vi "PhaseCompensation.vi"(1 "error out 2":errorcluster, 2 "Phase  Compensation":dbl) -> (0 "error out":errorcluster)   [LabVIEW 2011]
uses:
  C:/Entwicklungsdaten/Aktuell/Source/LV Source/arcoptix/LCDriver.dll
  Entwicklungsdaten/Aktuell/Source/LV Source/arcoptix/LCDriver.dll
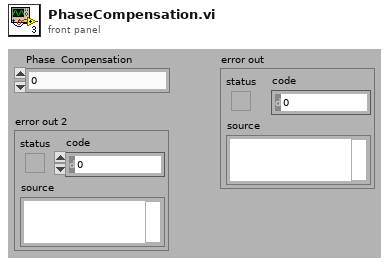
[diagram p1: front panel]
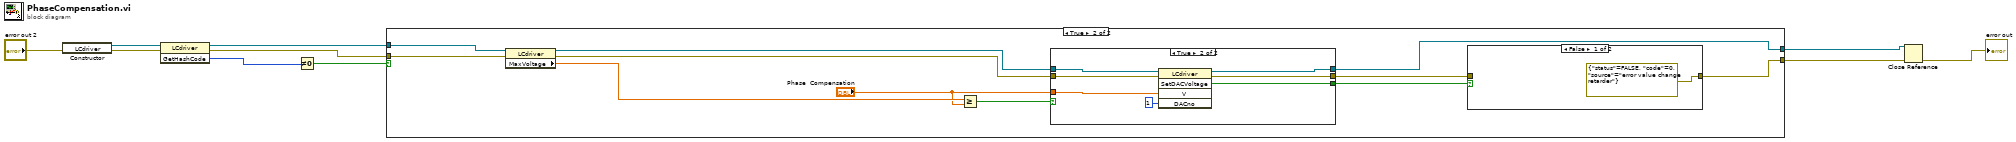
[diagram p0: block diagram]
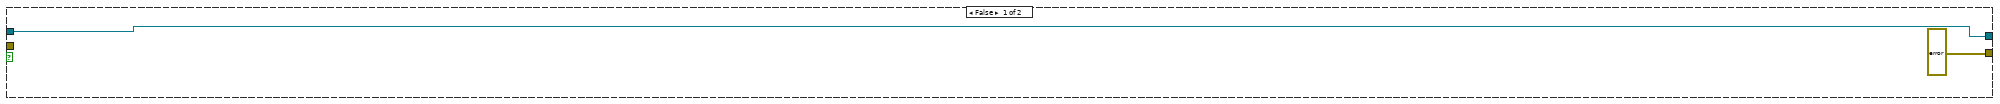
[diagram p2: hidden frame]
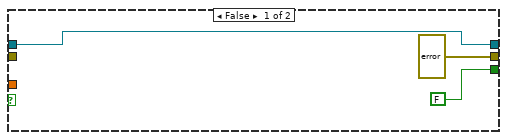
[diagram p4: hidden frame]
diagram:
  n1 = constructor class="LCdriver"(error in="error out 2") -> (reference out=w8:refnum<k24>, error out=w6:errorcluster)  [unwired: 2 in, 1 out]
  n2 = invoke class="LCdriver" method="GetHashCode"(reference=w8, error in=w6) -> (reference out=w7:refnum<k24>, error out=w5:errorcluster, "GetHashCode"=w3:i32)  [unwired: 1 in]
  n3 = Not Equal To 0?(x=w3) -> (x != 0?=w4:bool)
  n4 = case shown="True" w4 {
    tunnel: [errorcluster {"status"=FALSE, "code"=0, "source"="Error Methode ArcOptix"} ("error out") w14] -> w10
    tunnel: [w12 w21] -> w9
    tunnel: w7 -> [w12 w23]
    tunnel: w5 -> [_ w22]
    frame False {
    }
    frame True {
      n5 = property class="LCdriver"(reference=w23, error in=w22) -> (reference out=w20:refnum<k24>, error out=w19:errorcluster, "MaxVoltage"=w18:dbl)
      n6 = Greater Or Equal?(x=w18, y="Phase  Compensation") -> (x >= y?=w17:bool)
      n7 = case shown="True" w17 {
        tunnel: [w27 w34] -> w21
        tunnel: [errorcluster {"status"=FALSE, "code"=0, "source"="voltage to high, must be under 8,8volt"} ("error out") w33] -> w15
        tunnel: w20 -> [w27 w32]
        tunnel: w19 -> [_ w31]
        tunnel: [FALSE ("SetDACVoltage") w30] -> w13
        tunnel: "Phase  Compensation" -> [_ w29]
        frame False {
        }
        frame True {
          n8 = invoke class="LCdriver" method="SetDACVoltage"(reference=w32, error in=w31, "V"=w29, "DACno"=u8 1) -> (reference out=w34:refnum<k24>, error out=w33:errorcluster, "SetDACVoltage"=w30:bool)  [unwired: 1 in, 2 out]
        }
      }
      n9 = case shown="False" w13 {
        tunnel: w15 -> [_ w25]
        tunnel: [errorcluster {"status"=FALSE, "code"=0, "source"="error value change retarder"} ("error out") w25] -> w14
        frame False {
        }
        frame True {
        }
      }
    }
  }
  n10 = Close Reference(reference=w9, error in (no error)=w10) -> (error out=→"error out":errorcluster)
